vi "Done Glyph.vi"(8 "error in (no error)":errorcluster, 11 "glyph ref in":i64) -> (0 "error out":errorcluster)   [LabVIEW 2023, in "Freetype Drawer.lvlib"]
uses:
  Freetype Drawer.lvlib
  libfreetype.dll
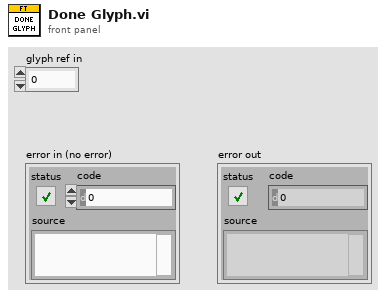
[diagram p1: front panel]
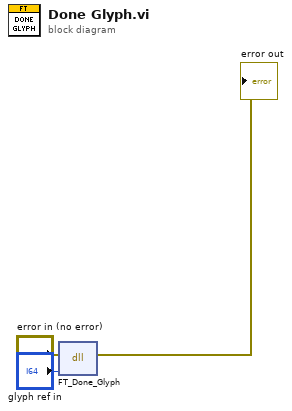
[diagram p0: block diagram]
diagram:
  n1 = dll-call lib="E:/Labview/LV 2023/Libs/LV Symbol/Freetype Drawer/libfreetype.dll" fn="FT_Done_Glyph"(error in="error in (no error)", "glyph in"="glyph ref in") -> (error out=→"error out":errorcluster)  [unwired: 4 in, 1 out]
